vi "Fast_seq_init.vi"(0 "FPGA Ref":T8, 1 "Ramp?":bool=TRUE, 2 "Fast sequence parameters 2":T7 {"fastseq"."DAC"."DAC offset" min=-1 max=0.5; "fastseq"."DAC"."FastChanNum" max=15 step=1; "fastseq"."slot#" max=4095}) -> ()   [LabVIEW 2013]
uses:
  fpga-bitfile-ref.ctl
  sequence slot/slot-use.ctl
  sequence slot/triggers.ctl
  sequence slot/DAC.ctl
  sequence slot/DAC_fastseq-offset.ctl
  sequence slot/timing.ctl
  sequence slot/jump.ctl
  sequence slot/data.ctl
  sequence slot/slot.xctl
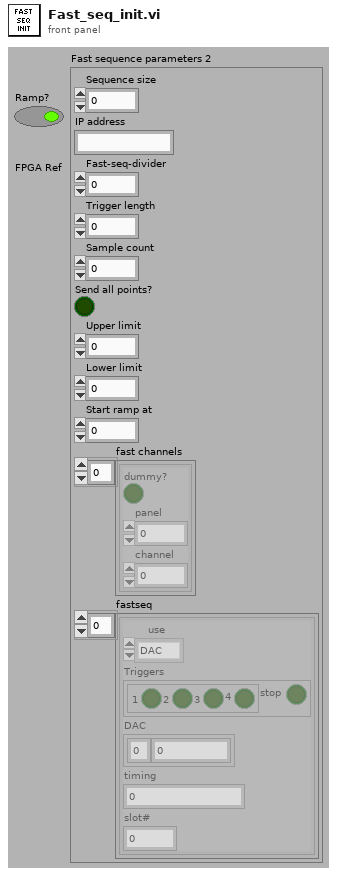
[diagram p1: front panel]
types:
  T1 = typedef "slot-use.ctl" = enum8{"DAC", "timing", "triggers", "jump"}
  T2 = typedef "triggers.ctl" = cluster{"triggers":cluster{"1":bool, "2":bool, "3":bool, "4":bool}, "stop":bool}
  T3 = typedef "DAC.ctl" = cluster{"FastChanNum":u8, "DAC offset":T4}
  T4 = typedef "DAC_fastseq-offset.ctl" = sgl
  T5 = typedef "timing.ctl" = sgl
  T6 = typedef "jump.ctl" = u16
  T7 = cluster{"Sequence size":u64, "IP address":string, "Fast-seq-divider":u64, "Trigger length":u64, "Sample count":u64, "Send all points?":bool, "Upper limit":dbl, "Lower limit":dbl, "Start ramp at":u64, "fast channels":cluster{"dummy?":bool, "panel":u8, "channel":u8}[], "fastseq":cluster{"use":T1, "Triggers":T2, "DAC":T3, "timing":T5, "slot#":T6}[]}
  T8 = typedef "fpga-bitfile-ref.ctl" = refnum<k20>
  T9 = cluster{"dummy?":bool, "panel":u8, "channel":u8}[]
  T10 = cluster{"use":T1, "Triggers":T2, "DAC":T3, "timing":T5, "slot#":T6}[]
  T11 = enum16{"stop", "set divider", "unset ramp mode", "unset stop count", "set pulse lenght", "set ramp", "start"}
  T12 = typedef "slot.xctl/data.ctl" = cluster{"use":T1, "Triggers":T2, "DAC":T3, "timing":T5, "slot#":T6}
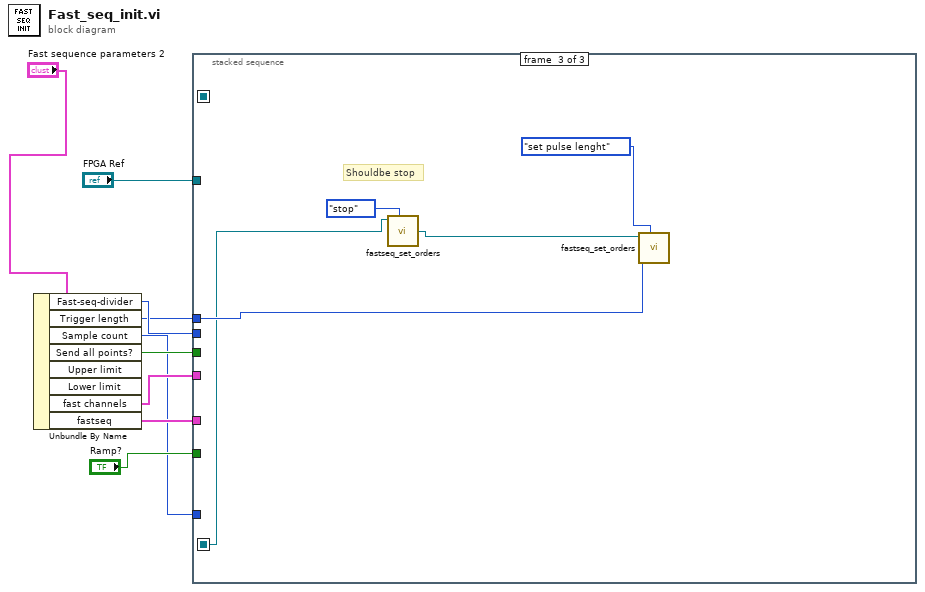
[diagram p0: block diagram]
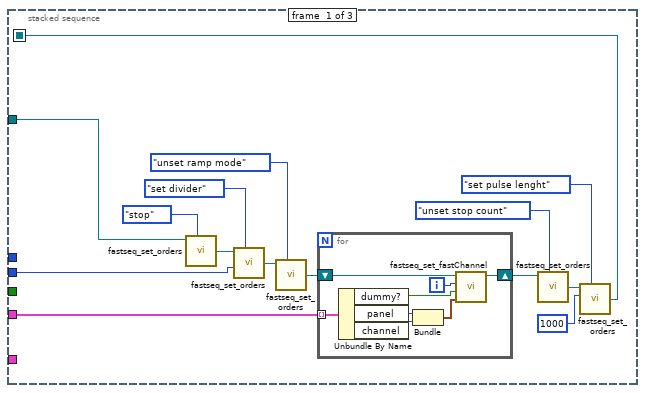
[diagram p2: hidden frame]
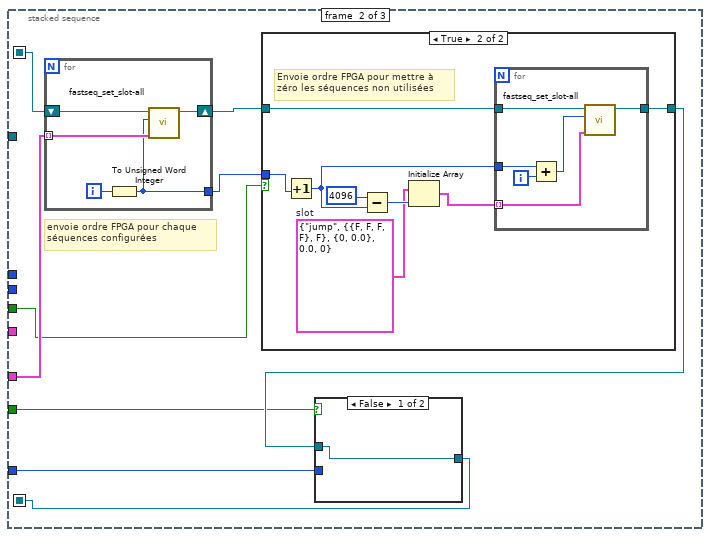
[diagram p3: hidden frame]
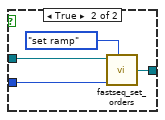
[diagram p4: hidden frame]
diagram:
  n1 = Unbundle By Name("Fast sequence parameters 2") -> ("Fast-seq-divider"=w9:u64, "Trigger length"=w3:u64, "Sample count"=w2:u64, "Send all points?"=w5:bool, "fast channels"=w8:T9, "fastseq"=w6:T10)  [unwired: 2 out]
  n2 = stacked-sequence {
    seq-local: [w10 _ _] -> [_ w34 _]
    seq-local: [_ w33 _] -> [_ _ w68]
    tunnel: w9 -> [w13 _ _]
    tunnel: w8 -> [w12 _ _]
    tunnel: "FPGA Ref" -> [w11 _ _]
    tunnel: w6 -> [_ w41 _]
    tunnel: w5 -> [_ w40 _]
    tunnel: "Ramp?" -> [_ w36 _]
    tunnel: w3 -> [_ _ w70]
    tunnel: w2 -> [_ w35 _]
    frame #0 {
      n3 = call "fastseq_set_orders.vi"("FPGA VI Reference In"=w11, "Enum"=T11."stop") -> ("FPGA VI Reference Out"=w17:T8)  [unwired: 3 in]
      n4 = call "fastseq_set_orders.vi"("FPGA VI Reference In"=w17, "divider"=w13, "Enum"=T11."set divider") -> ("FPGA VI Reference Out"=w20:T8)  [unwired: 2 in]
      n5 = call "fastseq_set_orders.vi"("FPGA VI Reference In"=w20, "Enum"=T11."unset ramp mode") -> ("FPGA VI Reference Out"=w14:T8)  [unwired: 3 in]
      n6 = for {
        tunnel: w12 -> [w31] mode=indexing
        shift-right: [w32] -> w22
        shift-left: w14 -> [w25]
        i -> [w26]
        n7 = Unbundle By Name(w31) -> ("dummy?"=w30:bool, "panel"=w27:u8, "channel"=w28:u8)
        n8 = Bundle("panel"=w27, "channel"=w28) -> (w29:cluster{"panel":u8, "channel":u8})  [unwired: 1 out]
        n9 = call "fastseq_set_fastChannel.vi"("pan-channel"=w29, "is dummy?"=w30, "fast chan number"=w26, "FPGA VI Reference In"=w25) -> ("FPGA VI Reference Out"=w32:T8)  [unwired: 7 out]
      }
      n10 = call "fastseq_set_orders.vi"("FPGA VI Reference In"=w22, "Enum"=T11."unset stop count") -> ("FPGA VI Reference Out"=w23:T8)  [unwired: 3 in]
      n11 = call "fastseq_set_orders.vi"("FPGA VI Reference In"=w23, "pulse length"=u16 1000, "Enum"=T11."set pulse lenght") -> ("FPGA VI Reference Out"=w10:T8)  [unwired: 2 in]
    }
    frame #1 {
      # "envoie ordre FPGA pour chaque\nséquences configurées"
      n12 = for {
        tunnel: w41 -> [w66] mode=indexing
        tunnel: [w64] -> w38
        shift-right: [w62] -> w39
        shift-left: w34 -> [w63]
        i -> [w65]
        n13 = To Unsigned Word Integer(number=w65) -> (unsigned 16bit integer=w64:u16)
        n14 = call "fastseq_set_slot-all.vi"("slot"=w66, "slot number"=w64, "FPGA VI Reference In"=w63) -> ("FPGA VI Reference Out"=w62:T8)  [unwired: 3 in, 5 out]
      }
      n15 = case shown="True" w40 {
        tunnel: w39 -> [w47 w50]
        tunnel: w38 -> [_ w49]
        tunnel: [w47 w48] -> w37
        frame False {
        }
        frame True {
          w51 = T12 {"use"=enum."jump", "Triggers"={"triggers"={"1"=FALSE, "2"=FALSE, "3"=FALSE, "4"=FALSE}, "stop"=FALSE}, "DAC"={"FastChanNum"=0, "DAC offset"=0.0}, "timing"=0.0, "slot#"=0}  # slot
          # "Envoie ordre FPGA pour mettre à \nzéro les séquences non utilisées"
          n16 = Increment(x=w49) -> (x+1=w54:u16)
          n17 = Subtract(x=u16 4096, y=w54) -> (x-y=w52:u16)
          n18 = Initialize Array(w51, w52) -> (w55:T12[])
          n19 = for {
            tunnel: [w61] -> w48
            tunnel: w55 -> [w60] mode=indexing
            tunnel: w54 -> [w58]
            tunnel: w50 -> [w56]
            i -> [w59]
            n20 = Add(x=w58, y=w59) -> (x+y=w57:i32)
            n21 = call "fastseq_set_slot-all.vi"("slot"=w60, "slot number"=w57, "FPGA VI Reference In"=w56) -> ("FPGA VI Reference Out"=w61:T8)  [unwired: 2 in, 6 out]
          }
        }
      }
      n22 = case shown="False" w36 {
        tunnel: w37 -> [w42 w45]
        tunnel: w35 -> [_ w44]
        tunnel: [w42 w43] -> w33
        frame False {
        }
        frame True {
          n23 = call "fastseq_set_orders.vi"("FPGA VI Reference In"=w45, "sample count"=w44, "Enum"=T11."set ramp") -> ("FPGA VI Reference Out"=w43:T8)  [unwired: 2 in]
        }
      }
    }
    frame #2 {
      # "Shouldbe stop"
      n24 = call "fastseq_set_orders.vi"("FPGA VI Reference In"=w68, "Enum"=T11."stop") -> ("FPGA VI Reference Out"=w67:T8)  [unwired: 3 in]
      n25 = call "fastseq_set_orders.vi"("FPGA VI Reference In"=w67, "pulse length"=w70, "Enum"=T11."set pulse lenght") -> ()  [unwired: 2 in, 1 out]
    }
  }
